vi "set tilt degs.vi"(8 "error in (no error)":errorcluster, 10 "angle":i32, 11 "index":i32) -> (0 "error out":errorcluster, 3 "function return":i32)   [LabVIEW 2017, in "libfreenect.lvlib"]
doc: "EXPORT int freenect_lv_set_tilt_degs(int angle, int index);"
uses:
  libfreenect.lvlib
  freenect_lv.dll
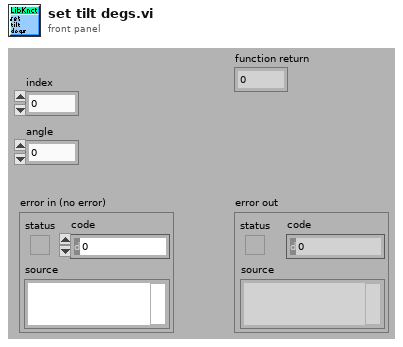
[diagram p1: front panel]
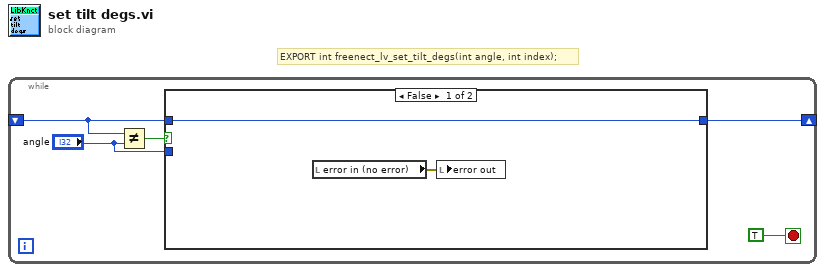
[diagram p0: block diagram]
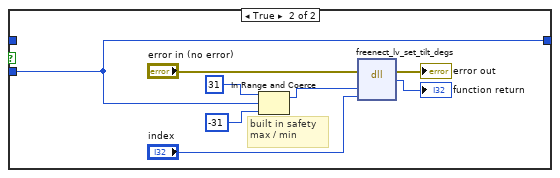
[diagram p2: hidden frame]
diagram:
  # "EXPORT int freenect_lv_set_tilt_degs(int angle, int index);"
  n1 = while {
    shift-right: [w1] -> _
    shift-left: _ -> [w3]
    stop <- TRUE stop-if-true
    n2 = Not Equal?(x=w3, y="angle") -> (x != y?=w4:bool)
    n3 = case shown="False" w4 {
      tunnel: "angle" -> [_ w8]
      tunnel: w3 -> [w7 _]
      tunnel: [w7 w8] -> w1
      frame False {
        n4 = local read "error in (no error)"() -> (w6:errorcluster)
        n5 = local write "error out"(w6) -> ()
      }
      frame True {
        # "built in safety max / min"
        n6 = In Range and Coerce(upper limit=31, x=w8, lower limit=-31) -> (coerced(x)=w15:i32)  [unwired: 1 out]
        n7 = dll-call lib="C:/Users/Mats/Desktop/Bacheler prosjekt/Labview/Occupancy Grid Map Code - With model/freenect_lv.*" fn="freenect_lv_set_tilt_degs"(error in="error in (no error)", "angle"=w15, "index"="index") -> (error out=→"error out":errorcluster, →"function return":i32)  [unwired: 4 in, 1 out]
      }
    }
  }
